vi "Search Object List.vi"(10 "Object ID":u8 format="%x", 11 "Objects":T1[](array[typedef]) {"Object ID" format="%x"}) -> (2 "Object":T1 {"Object ID" format="%x"}, 3 "Found?":bool, 5 "Index":i32)   [LabVIEW 2015, in "Modbus Library.lvlib" / "Device Data Model.lvclass"]
doc: "This VI looks for a specific object in the full list."
uses:
  Device Data Model.lvclass
  Identification Parameters.ctl
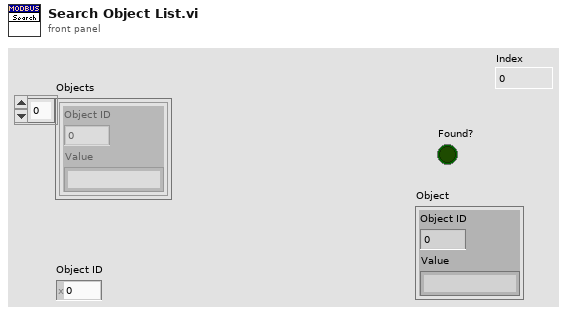
[diagram p1: front panel]
types:
  T1 = typedef "Modbus Library.lvlib/Device Data Model.lvclass/Identification Parameters.ctl" = cluster{"Object ID":u8, "Value":string}
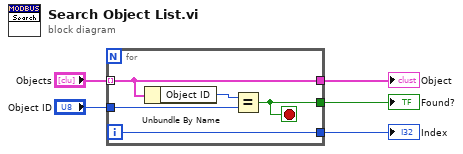
[diagram p0: block diagram]
diagram:
  n1 = for {
    tunnel: "Objects" -> [w8] mode=indexing
    tunnel: "Object ID" -> [w9]
    tunnel: [w8] -> w3
    tunnel: [w7] -> w2
    tunnel: [w6] -> w1
    i -> [w6]
    stop <- w7 stop-if-true
    n2 = Unbundle By Name(w8) -> ("Object ID"=w10:u8)
    n3 = Equal?(x=w10, y=w9) -> (x = y?=w7:bool)
  }
  "Found?" <- w2
  "Object" <- w3
  "Index" <- w1
